vi "项操作.vi"(8 "error in (no error)":errorcluster caption="错误输入（无错误）", 9 "Cell Position":T1, 10 "MCListbox引用句柄":refnum<vi>, 11 "Copy 输入":refnum<class "Copy.lvclass">) -> (0 "error out":errorcluster caption="错误输出", 3 "Copy 输出":refnum<class "Copy.lvclass">)   [LabVIEW 2016, in "Copy.lvclass"]
uses:
  Copy.lvclass
  <vilib>/Utility/miscctls.llb/LVRowAndColumnTypeDef.ctl
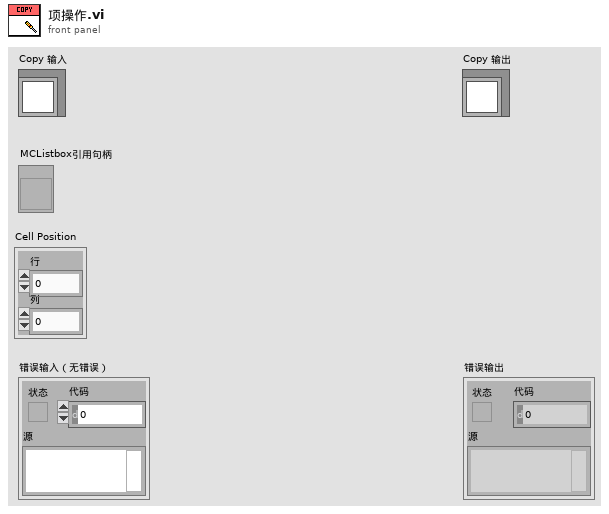
[diagram p1: front panel]
types:
  T1 = typedef "LVRowAndColumnTypeDef.ctl" = cluster{"Row":i32, "Column":i32}
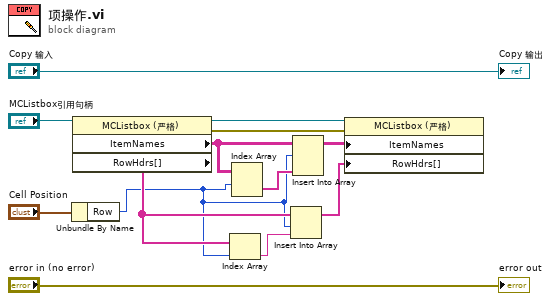
[diagram p0: block diagram]
diagram:
  n1 = Unbundle By Name("Cell Position") -> ("Row"=w1:i32)
  n2 = property class="MCListbox (严格)"(reference="MCListbox引用句柄") -> (reference out=w10:refnum<vi>, error out=w9:errorcluster, "ItemNames"=w7:string[][], "RowHdrs[]"=w4:string[])  [unwired: 1 in]
  n3 = Index Array(array=w4, index=w1) -> (element=w5:string)
  n4 = Index Array(array=w7, index (row)=w1) -> (element=w8:string[])  [unwired: 1 in]
  n5 = Insert Into Array(array=w4, index=w1, new element=w5) -> (w3:string[])
  n6 = Insert Into Array(array=w7, index (row)=w1, new element=w8) -> (w6:string[][])  [unwired: 1 in]
  n7 = property class="MCListbox (严格)"(reference=w10, error in=w9, "ItemNames"=w6, "RowHdrs[]"=w3) -> ()  [unwired: 2 out]
  "error out" <- "error in (no error)"
  "Copy 输出" <- "Copy 输入"
